vi "Populate Run-Time Menu.vi"(8 "error in (no error)":errorcluster, 11 "Menu in":refnum<k9>) -> (0 "error out":errorcluster)   [LabVIEW 2020, in "Execution UI.lvclass"]
uses:
  Execution UI.lvclass
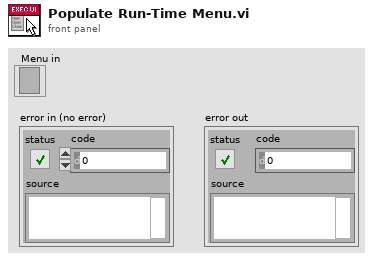
[diagram p1: front panel]
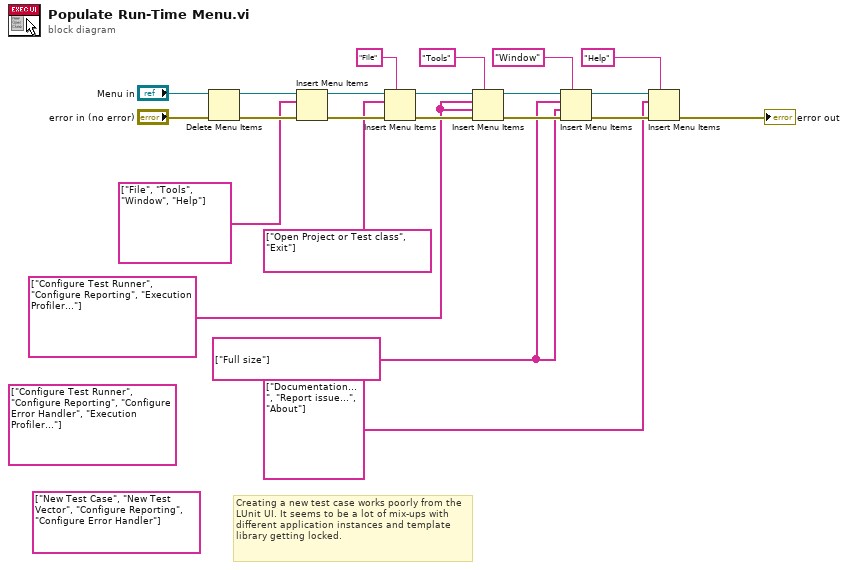
[diagram p0: block diagram]
diagram:
  (unwired) string[] ["Configure Test Runner", "Configure Reporting", "Configure Error Handler", "Execution Profiler..."] ("item names")
  (unwired) string[] ["New Test Case", "New Test Vector", "Configure Reporting", "Configure Error Handler"] ("item names")
  w1 = string[] ["Full size"] ("item names")
  w2 = string[] ["Configure Test Runner", "Configure Reporting", "Execution Profiler..."] ("item names")
  # "Creating a new test case works poorly from the LUnit UI. It seems to be a lot of mix-ups with different application instances and template library getting locked."
  n1 = Delete Menu Items(6:"error in (no error)", 9:"Menu in") -> (0:w19:errorcluster, 3:w21:refnum<k9>)  [unwired: 2 in]
  n2 = Insert Menu Items(6:w19, 8:string[] ["File", "Tools", "Window", "Help"] ("item names"), 9:w21) -> (0:w16:errorcluster, 3:w17:refnum<k9>)  [unwired: 3 in, 1 out]
  n3 = Insert Menu Items(5:"File" ("menu tag"), 6:w16, 8:string[] ["Open Project or Test class", "Exit"] ("item names"), 9:w17) -> (0:w10:errorcluster, 3:w9:refnum<k9>)  [unwired: 2 in, 1 out]
  n4 = Insert Menu Items(5:"Tools", 6:w10, 7:w2, 8:w2, 9:w9) -> (0:w11:errorcluster, 3:w8:refnum<k9>)  [unwired: 1 in, 1 out]
  n5 = Insert Menu Items(5:"Window", 6:w11, 7:w1, 8:w1, 9:w8) -> (0:w12:errorcluster, 3:w7:refnum<k9>)  [unwired: 1 in, 1 out]
  n6 = Insert Menu Items(5:"Help", 6:w12, 8:string[] ["Documentation...", "Report issue...", "About"] ("item names"), 9:w7) -> (0:→"error out":errorcluster)  [unwired: 2 in, 2 out]
